vi "LVClass_WavefrontCorrector Save current positions to file.vi"(0 "WavefrontCorrector in":refnum<class "WavefrontCorrector.lvclass">, 5 "filepath (*.wcs)":path, 11 "error in (no error)":errorcluster) -> (4 "WavefrontCorrector out":refnum<class "WavefrontCorrector.lvclass">, 15 "error out":errorcluster)   [LabVIEW 2020, in "WavefrontCorrector.lvclass"]
doc: "Perform a wavefront corrector action regarding its name.\n\n--------------------------------------------------------------------------------\n\n<B>correctorIn </B> : WavefrontCorrector object.\n<B>correctorOut </B> : WavefrontCorrector object.\n<B>feature_name </B> : Name of the action.\n<B>ErrorIn </B> : Error\n<B>ErrorOut </B> : Error\n\n--------------------------------------------------------------------------------"
uses:
  WavefrontCorrector.lvclass
  WavefrontCorrector.lvclass/WavefrontCorrector.ctl
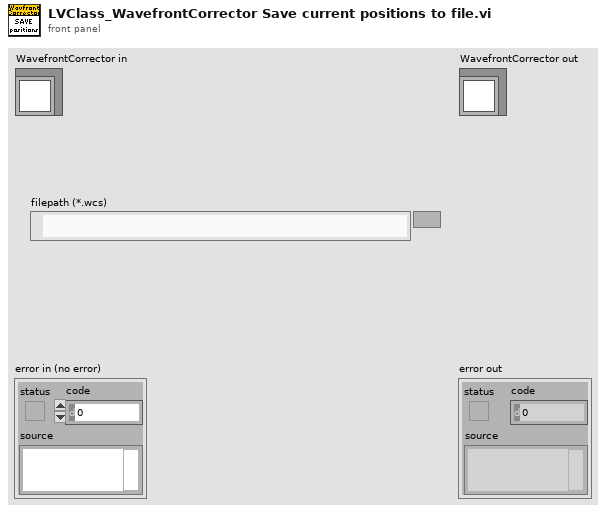
[diagram p1: front panel]
types:
  T1 = typedef "ClassID.ctl" = i64
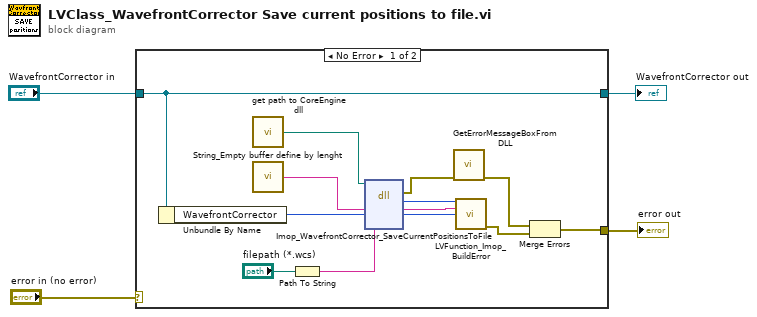
[diagram p0: block diagram]
diagram:
  n1 = case shown="No Error" "error in (no error)" {
    selector: "error in (no error)" -> [_ w19]
    tunnel: [w7 w19] -> w2
    tunnel: [w8 w18] -> w1
    tunnel: "WavefrontCorrector in" -> [w8 w18]
    frame No Error {
      n2 = Unbundle By Name(w8) -> ("WavefrontCorrector"=w11:T1)
      n3 = call "get path to CoreEngine dll.vi"() -> ("path to wavekit library"=w14:path)  [unwired: 14 in, 1 out]
      n4 = call "String_Empty buffer define by lenght.vi"() -> ("Empty buffer"=w17:string)  [unwired: 1 in]
      n5 = Path To String(path="filepath (*.wcs)") -> (string=w6:string)
      n6 = dll-call lib="D:/SOFTware/CoreEngine4_Suite/SVN_trunk/LV2011_interface/DLLs/c_interface_vc100.dll" fn="Imop_WavefrontCorrector_SaveCurrentPositionsToFile"(path in=w14, "message"=w17, "objet"=w11, "action_name"=w6) -> (error out=w13:errorcluster, "return type"=w15:i32, "message"=w16:string, "objet"=w5:i64)  [unwired: 3 in, 1 out]
      n7 = call "GetErrorMessageBoxFromDLL.vi"("error IN"=w13) -> ("error OUT"=w10:errorcluster)  [unwired: 10 in]
      n8 = call "LVFunction_Imop_BuildError.vi"("code"=w15, "String to Prepend to source (\"\")"=w16, "Adresse"=w5) -> ("error out"=w9:errorcluster)  [unwired: 12 in]
      n9 = Merge Errors(w10, w9) -> (w7:errorcluster)
    }
    frame Error {
    }
  }
  "error out" <- w2
  "WavefrontCorrector out" <- w1
